vi "SN_LinkData.vi"() -> ()   [LabVIEW 2019]
panel:
  in  "SN_CloseRef":refnum<vi>
  # "MainPanelSet"
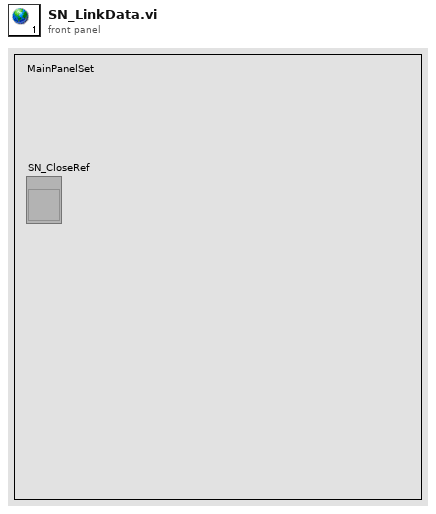
[diagram p1: front panel]
diagram:
